vi "VDT Channel.vi"(8 "error in (no error)":errorcluster, 11 "Node Ptr":T3 format="%.0x") -> (0 "error out":errorcluster)   [LabVIEW 2020, in "NI PXIe-4340 System Explorer.lvlib"]
uses:
  NI PXIe-4340 System Explorer.lvlib
  <vilib>/NI VeriStand/Custom Device API/Custom Device Item Ref.ctl
  Shared/Position_LVDT_Properties.ctl
  Shared/Position_RVDT_Properties.ctl
  Shared/Constants.vi
  <vilib>/NI VeriStand/Custom Device API/Get Item Property (Variant).vi
  <vilib>/NI VeriStand/Custom Device API/Get Item Property (Double).vi
  <vilib>/NI VeriStand/Custom Device API/Get Item Property (I32).vi
  <vilib>/NI VeriStand/Custom Device API/Set Item Property (I32).vi
  <vilib>/NI VeriStand/Custom Device API/Set Item Property (Double).vi
  <vilib>/NI VeriStand/Custom Device API/Set Item Property (Variant).vi
  <vilib>/NI VeriStand/Custom Device API/Custom Device API.lvlib
  Shared/NI PXIe-4340 Shared.lvlib
panel:
  out "Sensitivity Unit":string
  out "ExcValue Unit":string="Vrms"
  out "Freq Unit":string="Hz"
  out "Channel Unit 3":string
  out "Channel Unit 2":string
  out "Channel Unit":string
  in  "Initial Value":dbl
  in  "Measurement Type":i32(ring) items=["Position LVDT", "Position RVDT"]
  in  "Position_RVDT_Properties":T1={"Minimum Value"=-0.1, "Maximum Value"=0.1, "Excitation Source"=10200, "Excitation Wire Mode"=4, "Excitation Frequency"=2500.0, "Excitation Value"=1.0, "Units"=10146, "Sensitivity"=50.0, "Sensitivity Units"=12507, "Excitation Sense"=16095} {"Sensitivity Units" items=["mVolts/Volt/Degree"=12507, "mVolts/Volt/Radian"=12508]; "Units" items=["Degrees"=10146, "Radians"=10273, "From Custom Scale"=10065]; "Excitation Sense" items=["Local"=16095, "Remote"=16096]; "Excitation Source" items=["Internal"=10200, "External"=10167, "None"=10230]; "Excitation Wire Mode" items=["4-Wire"=4, "5-Wire"=5, "6-Wire"=6]}
  out "Physical Channel":string
  in  "Position_LVDT_Properties":T2={"Minimum Value"=-0.1, "Maximum Value"=0.1, "Excitation Source"=10200, "Excitation Wire Mode"=4, "Excitation Frequency"=2500.0, "Excitation Value"=1.0, "Units"=10219, "Sensitivity"=50.0, "Sensitivity Units"=12506, "Excitation Sense"=16095} {"Excitation Sense" items=["Local"=16095, "Remote"=16096]; "Excitation Source" items=["Internal"=10200, "External"=10167, "None"=10230]; "Excitation Wire Mode" items=["4-Wire"=4, "5-Wire"=5, "6-Wire"=6]; "Units" items=["Meters"=10219, "Inches"=10379, "From Custom Scale"=10065]; "Sensitivity Units" items=["mVolts/Volt/mMeter"=12506, "mVolts/Volt/0.001 Inch"=12505]}
  in  "Header":cluster{"Section Name":string}={"Section Name"="Custom Device Item Settings"}
  in  "Description":string
  in  "Name":string
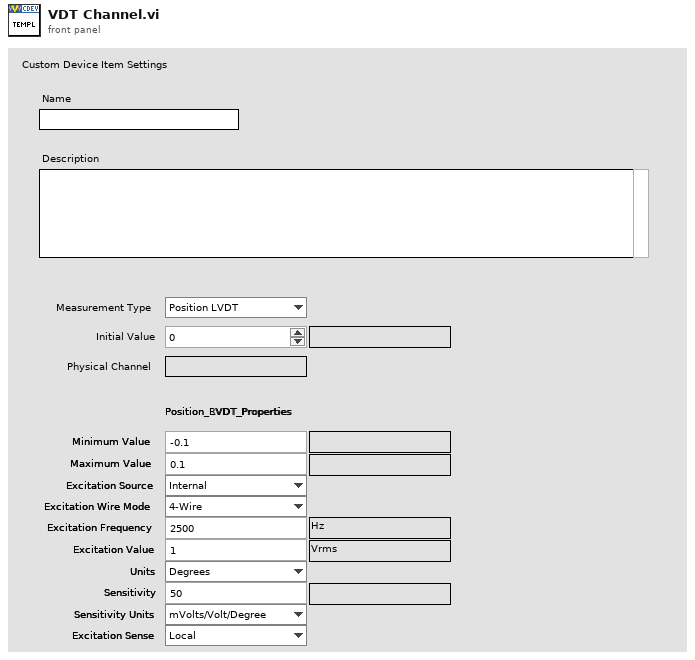
[diagram p1: front panel]
types:
  T1 = typedef "NI PXIe-4340 Shared.lvlib/Position_RVDT_Properties.ctl" = cluster{"Minimum Value":dbl, "Maximum Value":dbl, "Excitation Source":i32, "Excitation Wire Mode":i32, "Excitation Frequency":dbl, "Excitation Value":dbl, "Units":i32, "Sensitivity":dbl, "Sensitivity Units":i32, "Excitation Sense":i32}
  T2 = typedef "NI PXIe-4340 Shared.lvlib/Position_LVDT_Properties.ctl" = cluster{"Minimum Value":dbl, "Maximum Value":dbl, "Excitation Source":i32, "Excitation Wire Mode":i32, "Excitation Frequency":dbl, "Excitation Value":dbl, "Units":i32, "Sensitivity":dbl, "Sensitivity Units":i32, "Excitation Sense":i32}
  T3 = typedef "Custom Device API.lvlib/Custom Device Item Ref.ctl" = u64
  T4 = typedef "Custom Device API.lvlib/Custom Device Item Info.ctl" = cluster{"Name":string, "Is Channel":bool, "GUID":string, "Is Waveform":bool}
  T5 = typedef "Custom Device API.lvlib/Custom Device Commands.ctl" = enum16{"Default", "Item renamed", "Shutdown", "Dynamic button pressed"}
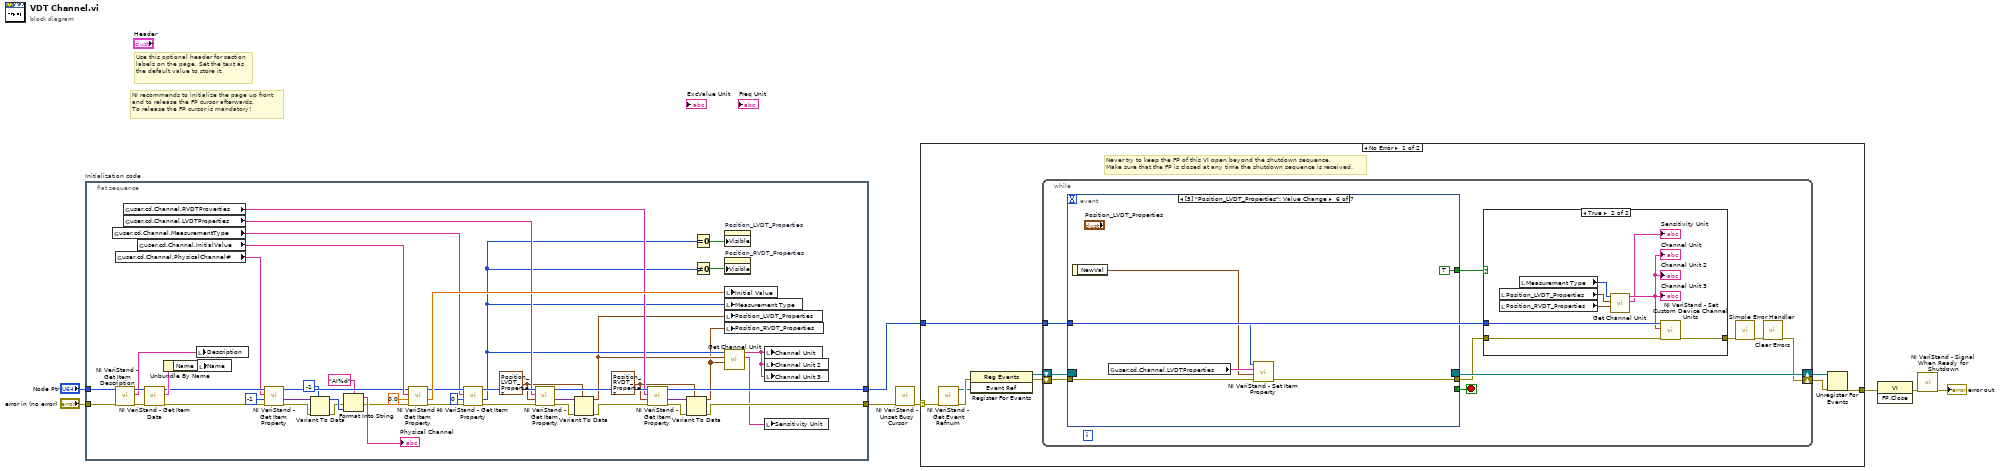
[diagram p0: block diagram]
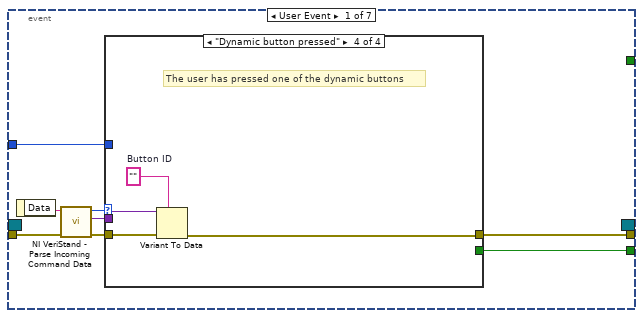
[diagram p3: hidden frame]
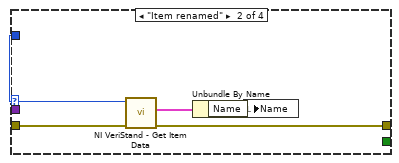
[diagram p5: hidden frame]
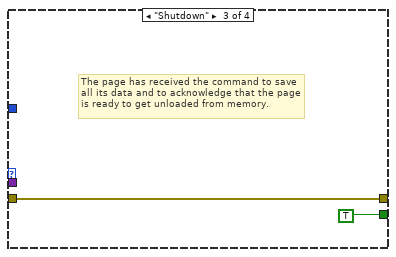
[diagram p6: hidden frame]
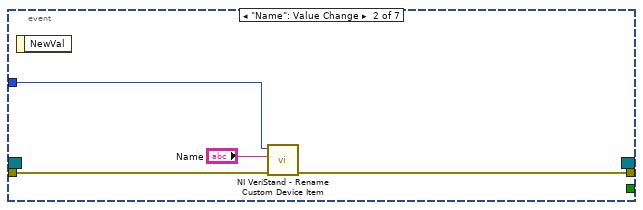
[diagram p7: hidden frame]
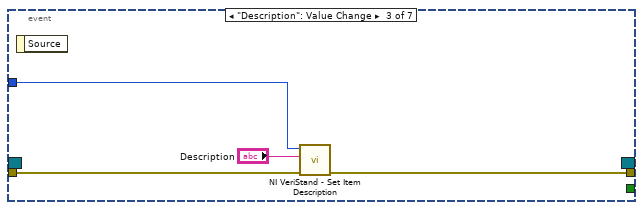
[diagram p8: hidden frame]
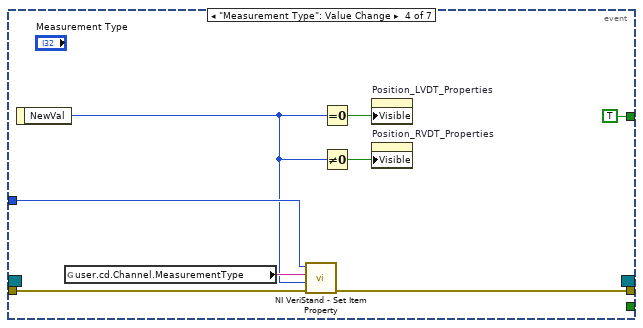
[diagram p9: hidden frame]
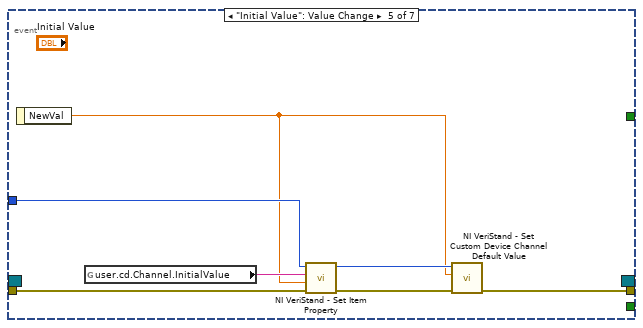
[diagram p10: hidden frame]
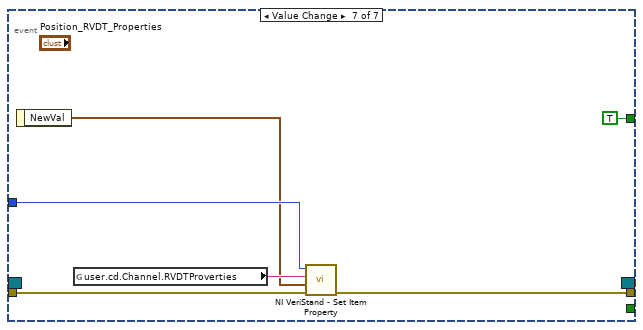
[diagram p11: hidden frame]
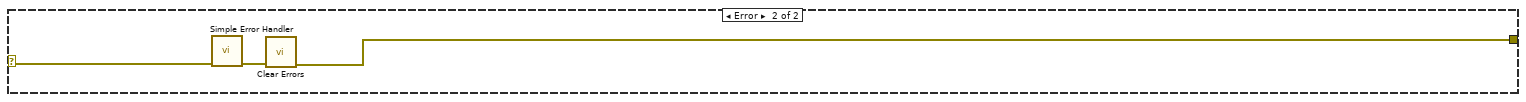
[diagram p12: hidden frame]
diagram:
  # "Use this optional header for section labels on the page. Set the text as the default value to store it."
  # "NI recommends to initialize the page up front\nand to release the FP cursor afterwards.\nTo release the FP cursor is mandatory!"
  n1 = flat-sequence "Initialization code" {
    tunnel: "error in (no error)" -> [w55]
    tunnel: "Node Ptr" -> [w54]
    tunnel: [w31] -> w4
    tunnel: [w30] -> w1
    frame #0 {
      w11 = T1 {"Minimum Value"=-70.0, "Maximum Value"=70.0, "Excitation Source"=10200, "Excitation Wire Mode"=4, "Excitation Frequency"=2500.0, "Excitation Value"=1.0, "Units"=10146, "Sensitivity"=50.0, "Sensitivity Units"=12507, "Excitation Sense"=16095} ("Position_RVDT_Properties")
      w34 = T2 {"Minimum Value"=-0.1, "Maximum Value"=0.1, "Excitation Source"=10200, "Excitation Wire Mode"=4, "Excitation Frequency"=2500.0, "Excitation Value"=1.0, "Units"=10219, "Sensitivity"=50.0, "Sensitivity Units"=12506, "Excitation Sense"=16095} ("Position_LVDT_Properties")
      n2 = global read "Constants.vi" "user.cd.Channel.MeasurementType"() -> (w45:string)
      n3 = global read "Constants.vi" "user.cd.Channel.PhysicalChannel#"() -> (w28:string)
      n4 = call <vilib>:"NI VeriStand - Get Item Description.vi"("error in (no error)"=w55, "Item Ref in"=w54) -> ("error out"=w52:errorcluster, "Description"=w53:string, "Item Ref out"=w56:T3)  [unwired: 7 out]
      n5 = global read "Constants.vi" "user.cd.Channel.RVDTProverties"() -> (w38:string)
      n6 = global read "Constants.vi" "user.cd.Channel.LVDTProperties"() -> (w40:string)
      n7 = global read "Constants.vi" "user.cd.Channel.InitialValue"() -> (w49:string)
      n8 = call <vilib>:"NI VeriStand - Get Item Data.vi"("error in (no error)"=w52, "Item Ref in"=w56) -> ("error out"=w27:errorcluster, "Item Info"=w51:T4, "Item Ref out"=w29:T3)  [unwired: 7 out]
      n9 = Unbundle By Name(w51) -> ("Name"=w50:string)
      n10 = local write "Description"(w53) -> ()
      n11 = local write "Name"(w50) -> ()
      n12 = call-poly <vilib>:"NI VeriStand - Get Item Property.vi"("error in (no error)"=w27, "Default Value"=-1, "Property Name"=w28, "Item Ref in"=w29) -> ("error out"=w22:errorcluster, "Value"=w25:variant, "Item Ref out"=w26:T3)  [unwired: 4 in, 1 out]
      n13 = Variant To Data(error in=w22, type=-1, Variant=w25) -> (data=w19:i32, error out=w17:errorcluster)
      n14 = Format Into String(format string="AI%d", error in=w17, w19) -> (resulting string=→"Physical Channel":string, error out=w16:errorcluster)  [unwired: 1 in]
      n15 = call-poly <vilib>:"NI VeriStand - Get Item Property.vi"("error in (no error)"=w16, "Default Value"=0.0, "Property Name"=w49, "Item Ref in"=w26) -> ("error out"=w43:errorcluster, "Value"=w47:dbl, "Item Ref out"=w46:T3)  [unwired: 4 in, 1 out]
      n16 = call-poly <vilib>:"NI VeriStand - Get Item Property.vi"("error in (no error)"=w43, "Default Value"=0, "Property Name"=w45, "Item Ref in"=w46) -> ("error out"=w41:errorcluster, "Value"=w14:i32, "Item Ref out"=w42:T3)  [unwired: 4 in, 1 out]
      n17 = call-poly <vilib>:"NI VeriStand - Get Item Property.vi"("error in (no error)"=w41, "Default Value"=w34, "Property Name"=w40, "Item Ref in"=w42) -> ("error out"=w36:errorcluster, "Value"=w35:variant, "Item Ref out"=w39:T3)  [unwired: 4 in, 1 out]
      n18 = Variant To Data(error in=w36, type=w34, Variant=w35) -> (data=w13:T2, error out=w37:errorcluster)
      n19 = call-poly <vilib>:"NI VeriStand - Get Item Property.vi"("error in (no error)"=w37, "Default Value"=w11, "Property Name"=w38, "Item Ref in"=w39) -> ("error out"=w33:errorcluster, "Value"=w32:variant, "Item Ref out"=w30:T3)  [unwired: 4 in, 1 out]
      n20 = Variant To Data(error in=w33, type=w11, Variant=w32) -> (data=w12:T1, error out=w31:errorcluster)
      n21 = Equal To 0?(x=w14) -> (x = 0?=w24:bool)
      n22 = Not Equal To 0?(x=w14) -> (x != 0?=w23:bool)
      n23 = property on="Position_LVDT_Properties" class="Clust (strict)"("Visible"=w24) -> ()  [unwired: 2 in, 2 out]
      n24 = property on="Position_RVDT_Properties" class="Clust (strict)"("Visible"=w23) -> ()  [unwired: 2 in, 2 out]
      n25 = local write "Initial Value"(w47) -> ()
      n26 = local write "Measurement Type"(w14) -> ()
      n27 = local write "Position_LVDT_Properties"(w13) -> ()
      n28 = local write "Position_RVDT_Properties"(w12) -> ()
      n29 = call "Get Channel Unit.vi"("Position_RVDT_Properties"=w12, "Position_LVDT_Properties"=w13, "Measurement Type"=w14) -> ("Sensitivity Unit"=w10:string, "Channel Unit"=w9:string)  [unwired: 7 in]
      n30 = local write "Channel Unit"(w9) -> ()
      n31 = local write "Channel Unit 2"(w9) -> ()
      n32 = local write "Channel Unit 3"(w9) -> ()
      n33 = local write "Sensitivity Unit"(w10) -> ()
    }
  }
  n34 = call <vilib>:"NI VeriStand - Unset Busy Cursor.vi"("error in (no error)"=w4) -> ("error out"=w3:errorcluster)  [unwired: 10 out]
  n35 = case shown="No Error" w3 {
    selector: w3 -> [w57 w142]
    tunnel: [w62 w140] -> w8
    tunnel: w1 -> [w58 _]
    frame No Error {
      # "Never try to keep the FP of this VI open beyond the shutdown sequence.\nMake sure that the FP is closed at any time the shutdown sequence is received."
      n36 = call <vilib>:"NI VeriStand - Get Event Refnum.vi"("error in (no error)"=w57) -> ("error out"=w65:errorcluster, "Event Ref"=w61:refnum<user-event>)  [unwired: 9 out]
      n37 = register-events(error in=w65, w61) -> (reference out=w59:refnum<event-registration>, error out=w60:errorcluster)  [unwired: 1 in]
      n38 = while {
        tunnel: w58 -> [w66]
        shift-right: [w70] -> w63
        shift-left: w60 -> [w74]
        shift-right: [w75] -> w64
        shift-left: w59 -> [w73]
        stop <- w72 stop-if-true
        n39 = event shown="[5] \"Position_LVDT_Properties\": Value Change" {
          selector: w73 -> [_ _ _ _ _ _ _]
          dyn-events: [_ _ _ _ _ _ _] -> w75
          timeout: _ -> [_ _ _ _ _ _ _]
          tunnel: w74 -> [w92 w108 w111 w120 w127 w133 w139]
          tunnel: [w88 _ _ _ _ _ _] -> w72
          tunnel: [w87 w107 w110 w117 w122 w132 w138] -> w67
          tunnel: w66 -> [w86 w106 w112 w116 w126 w131 w137]
          tunnel: [_ _ _ TRUE _ TRUE TRUE] -> w69
          event User Event {
            n40 = event-data() -> ("Data"=w91:string)  [unwired: 1 out]
            n41 = call <vilib>:"NI VeriStand - Parse Incoming Command Data.vi"("error in (no error)"=w92, "Incoming data"=w91) -> ("error out"=w90:errorcluster, "Outgoing data"=w85:variant, "Action"=w89:T5)  [unwired: 7 out]
            n42 = case shown="\"Dynamic button pressed\"" w89 {
              tunnel: w90 -> [w93 w98 w99 w104]
              tunnel: [_ _ TRUE _] -> w88
              tunnel: [w93 w95 w99 w101] -> w87
              tunnel: w86 -> [_ w97 _ _]
              tunnel: w85 -> [_ _ _ w103]
              frame "Default", Default {
              }
              frame "Item renamed" {
                n43 = call <vilib>:"NI VeriStand - Get Item Data.vi"("error in (no error)"=w98, "Item Ref in"=w97) -> ("error out"=w95:errorcluster, "Item Info"=w96:T4)  [unwired: 8 out]
                n44 = Unbundle By Name(w96) -> ("Name"=w94:string)
                n45 = local write "Name"(w94) -> ()
              }
              frame "Shutdown" {
                # "The page has received the command to save all its data and to acknowledge that the page is ready to get unloaded from memory."
              }
              frame "Dynamic button pressed" {
                w102 = ""  # Button ID
                # "The user has pressed one of the dynamic buttons"
                n46 = Variant To Data(error in=w104, type=w102, Variant=w103) -> (error out=w101:errorcluster)  [unwired: 1 out]
              }
            }
          }
          event "Name": Value Change {
            n47 = event-data() -> ()  [unwired: 2 out]
            n48 = call <vilib>:"NI VeriStand - Rename Custom Device Item.vi"("error in (no error)"=w108, "New Name"="Name", "Item Ref in"=w106) -> ("error out"=w107:errorcluster)  [unwired: 1 in, 7 out]
          }
          event "Description": Value Change {
            n49 = event-data() -> ()  [unwired: 2 out]
            n50 = call <vilib>:"NI VeriStand - Set Item Description.vi"("error in (no error)"=w111, "Description"="Description", "Item Ref in"=w112) -> ("error out"=w110:errorcluster)  [unwired: 8 out]
          }
          event "Measurement Type": Value Change {
            n51 = event-data() -> ("NewVal"=w114:i32)  [unwired: 1 out]
            n52 = global read "Constants.vi" "user.cd.Channel.MeasurementType"() -> (w115:string)
            n53 = call-poly <vilib>:"NI VeriStand - Set Item Property.vi"("error in (no error)"=w120, "Value"=w114, "Property Name"=w115, "Item Ref in"=w116) -> ("error out"=w117:errorcluster)  [unwired: 5 in, 2 out]
            n54 = Equal To 0?(x=w114) -> (x = 0?=w119:bool)
            n55 = Not Equal To 0?(x=w114) -> (x != 0?=w118:bool)
            n56 = property on="Position_LVDT_Properties" class="Clust (strict)"("Visible"=w119) -> ()  [unwired: 2 in, 2 out]
            n57 = property on="Position_RVDT_Properties" class="Clust (strict)"("Visible"=w118) -> ()  [unwired: 2 in, 2 out]
          }
          event "Initial Value": Value Change {
            n58 = event-data() -> ("NewVal"=w121:dbl)  [unwired: 1 out]
            n59 = global read "Constants.vi" "user.cd.Channel.InitialValue"() -> (w125:string)
            n60 = call-poly <vilib>:"NI VeriStand - Set Item Property.vi"("error in (no error)"=w127, "Value"=w121, "Property Name"=w125, "Item Ref in"=w126) -> ("error out"=w123:errorcluster, "Item Ref out"=w124:T3)  [unwired: 5 in, 1 out]
            n61 = call <vilib>:"NI VeriStand - Set Custom Device Channel Default Value.vi"("error in (no error)"=w123, "Default Value"=w121, "Channel Ref in"=w124) -> ("error out"=w122:errorcluster)  [unwired: 7 in, 1 out]
          }
          event Value Change {
            n62 = event-data() -> ("NewVal"=w129:T2)  [unwired: 1 out]
            n63 = global read "Constants.vi" "user.cd.Channel.LVDTProperties"() -> (w130:string)
            n64 = call-poly <vilib>:"NI VeriStand - Set Item Property.vi"("error in (no error)"=w133, "Value"=w129, "Property Name"=w130, "Item Ref in"=w131) -> ("error out"=w132:errorcluster)  [unwired: 5 in, 2 out]
          }
          event Value Change {
            n65 = event-data() -> ("NewVal"=w135:T1)  [unwired: 1 out]
            n66 = global read "Constants.vi" "user.cd.Channel.RVDTProverties"() -> (w136:string)
            n67 = call-poly <vilib>:"NI VeriStand - Set Item Property.vi"("error in (no error)"=w139, "Value"=w135, "Property Name"=w136, "Item Ref in"=w137) -> ("error out"=w138:errorcluster)  [unwired: 5 in, 2 out]
          }
        }
        n68 = case shown="True" w69 {
          tunnel: [w76 w82] -> w68
          tunnel: w67 -> [w76 w83]
          tunnel: w66 -> [_ w81]
          frame False {
          }
          frame True {
            n69 = local read "Position_RVDT_Properties"() -> (w84:T1)
            n70 = local read "Position_LVDT_Properties"() -> (w80:T2)
            n71 = local read "Measurement Type"() -> (w79:i32)
            n72 = call "Get Channel Unit.vi"("Position_RVDT_Properties"=w84, "Position_LVDT_Properties"=w80, "Measurement Type"=w79) -> ("Sensitivity Unit"=→"Sensitivity Unit":string, "Channel Unit"=w78:string)  [unwired: 7 in]
            "Channel Unit" <- w78
            "Channel Unit 2" <- w78
            "Channel Unit 3" <- w78
            n73 = call <vilib>:"NI VeriStand - Set Custom Device Channel Units.vi"("error in (no error)"=w83, "Units"=w78, "Channel Ref in"=w81) -> ("error out"=w82:errorcluster)  [unwired: 7 in, 1 out]
          }
        }
        n74 = call <vilib>:"Simple Error Handler.vi"("error in (no error)"=w68) -> ("error out"=w71:errorcluster)  [unwired: 1 in, 7 out]
        n75 = call <vilib>:"Clear Errors.vi"("error in (no error)"=w71) -> ("error out"=w70:errorcluster)  [unwired: 1 in, 5 out]
      }
      n76 = Unregister For Events(event registration refnum=w64, error in=w63) -> (error out=w62:errorcluster)
    }
    frame Error {
      n77 = call <vilib>:"Simple Error Handler.vi"("error in (no error)"=w142) -> ("error out"=w141:errorcluster)  [unwired: 1 in, 7 out]
      n78 = call <vilib>:"Clear Errors.vi"("error in (no error)"=w141) -> ("error out"=w140:errorcluster)  [unwired: 1 in, 5 out]
    }
  }
  n79 = invoke class="VI" method="FP.Close"(error in=w8) -> (error out=w7:errorcluster)  [unwired: 2 in, 2 out]
  n80 = call <vilib>:"NI VeriStand - Signal When Ready for Shutdown.vi"("error in (no error)"=w7) -> ("error out"=→"error out":errorcluster)  [unwired: 10 out]
